vi "LV_n_UDP_clients.vi"() -> ()   [LabVIEW 2020]
panel:
  in  "Open Multi Ports":bool
  in  "Open Single Port":bool
  in  "Send Test Image":bool
  in  "h":i32=10 min=1 max=5000 step=1
  in  "w":i32=1 min=1 max=5000 step=1
  out "Elaps ms":u32
  in  "Send Image":bool
  out "Path to Python script":path
  in  "Stop":bool
  out "Answer":string
  in  "Ping":bool
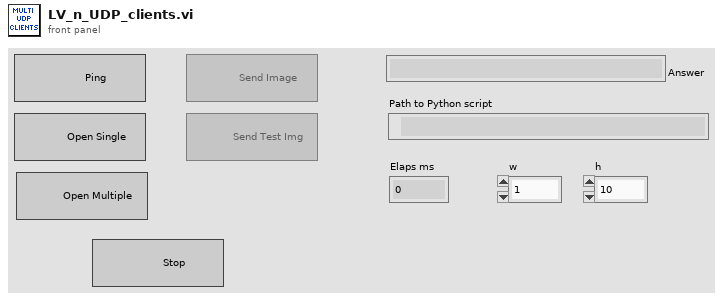
[diagram p1: front panel]
types:
  T1 = enum8{"Enabled", "Disabled", "Disabled and Grayed Out"}
  T2 = typedef "Image Type" = u32
  T3 = typedef "IMAQ Image.ctl" = refnum<image>
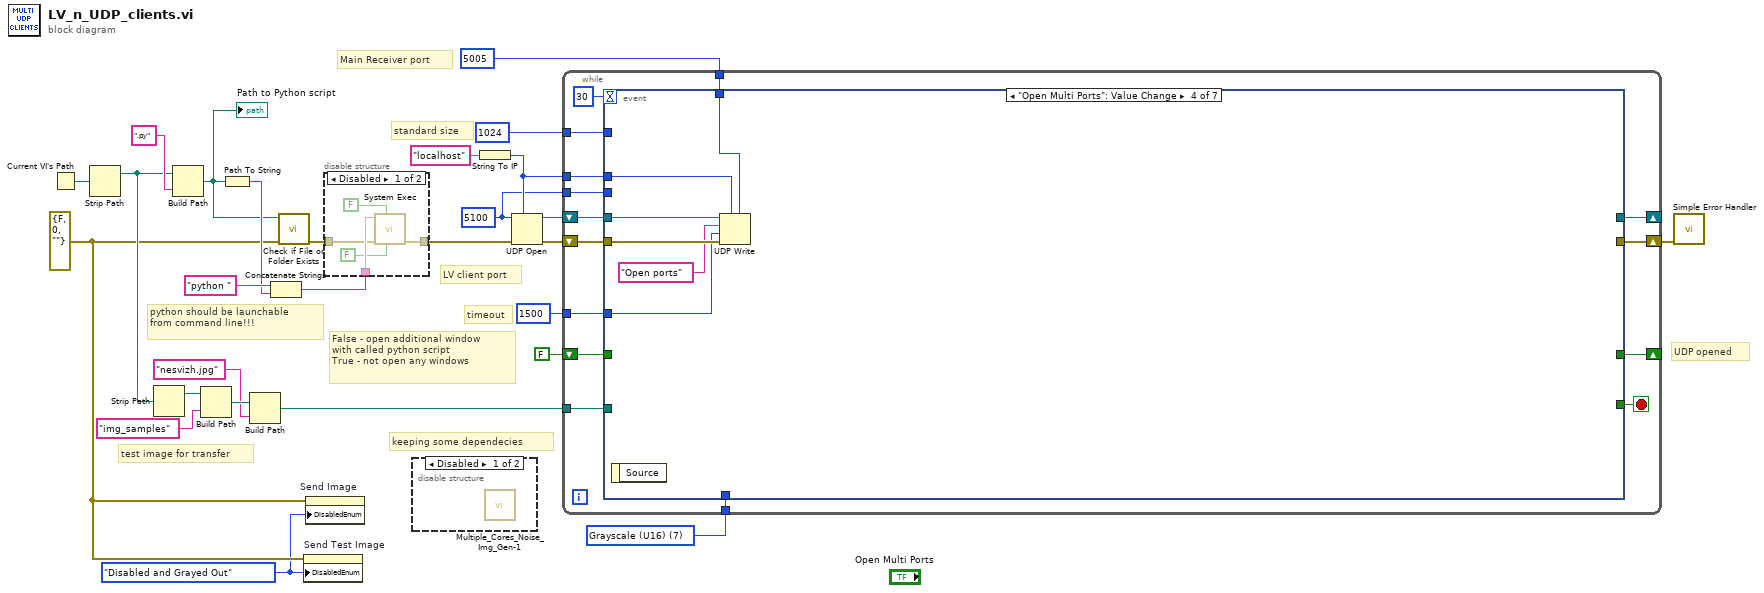
[diagram p0: block diagram]
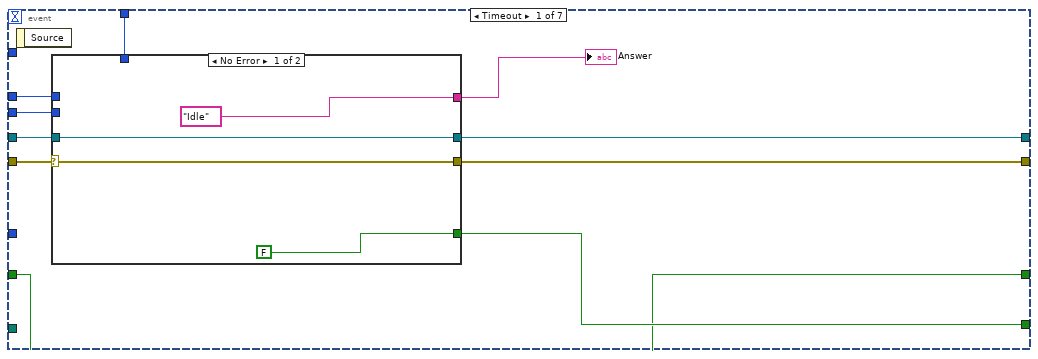
[diagram p4: hidden frame]
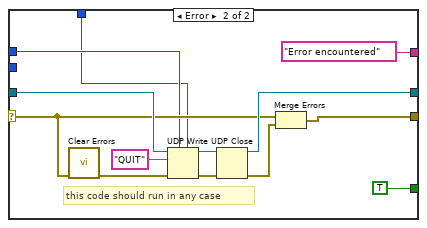
[diagram p5: hidden frame]
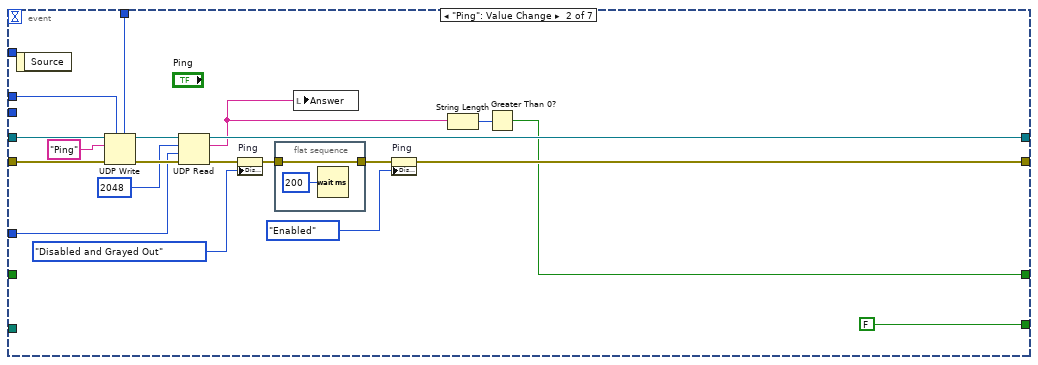
[diagram p6: hidden frame]
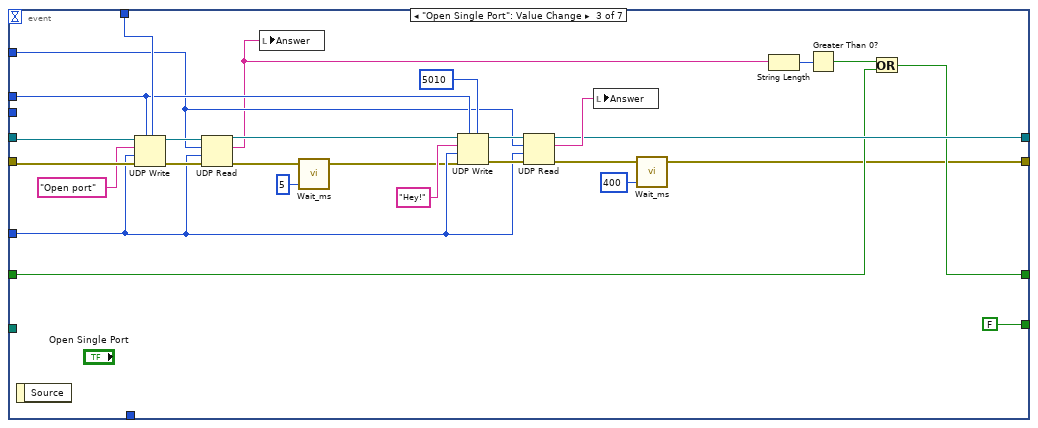
[diagram p7: hidden frame]
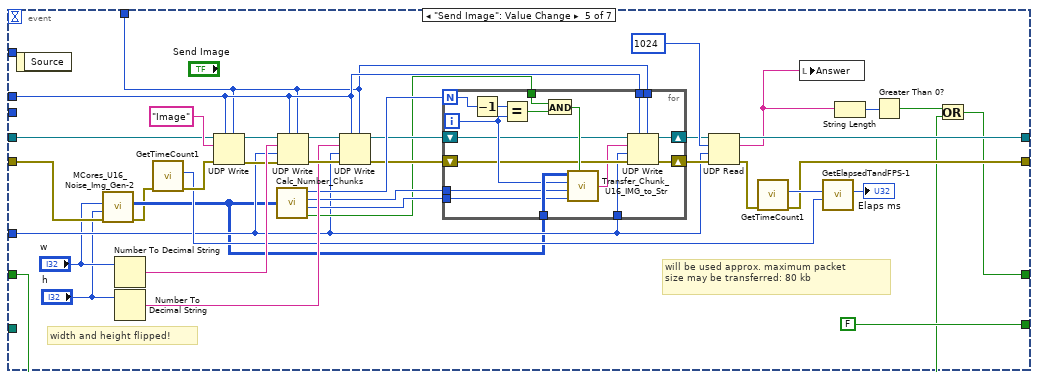
[diagram p8: hidden frame]
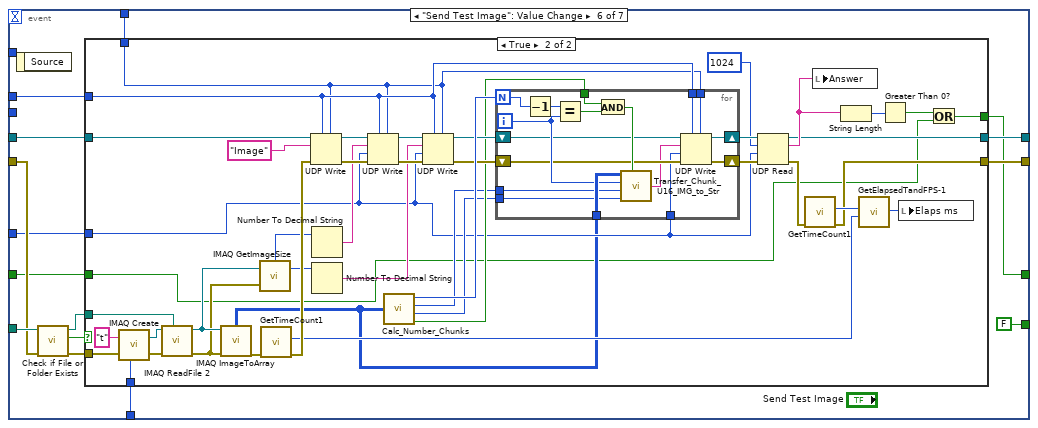
[diagram p9: hidden frame]
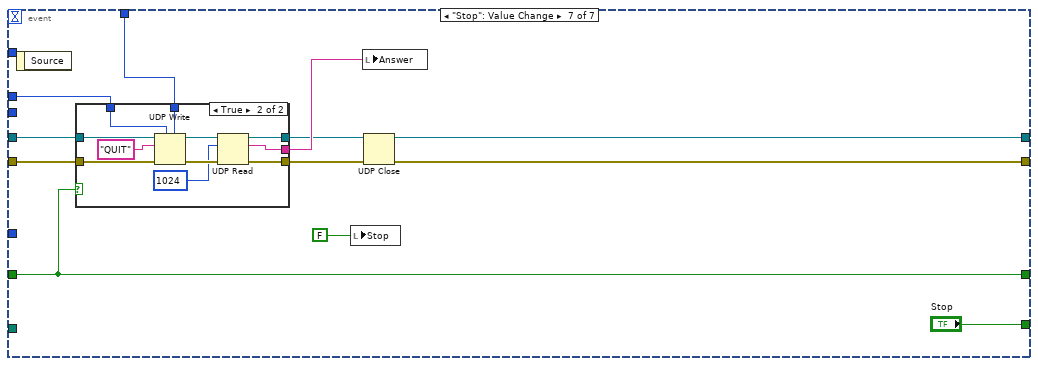
[diagram p11: hidden frame]
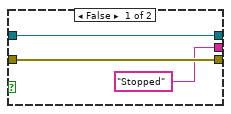
[diagram p12: hidden frame]
diagram:
  w3 = T1."Disabled and Grayed Out" ("Disabled")
  w5 = T2 7 items=["Grayscale (U8)", "Grayscale (I16)", "Grayscale (SGL)", "Complex (CSG)", "RGB (U32)", "HSL (U32)", "RGB (U64)", "Grayscale (U16)"] ("Image Type")
  w14 = u16 5100 ("remote port or service name")
  w4 = errorcluster {"status"=FALSE, "code"=0, "source"=""} ("error in (no error)")
  # "standard size"
  # "UDP opened"
  # "test image for transfer"
  # "keeping some dependecies"
  # "timeout"
  # "Main Receiver port"
  # "LV client port"
  # "False - open additional window\nwith called python script\nTrue - not open any windows"
  # "python should be launchable \nfrom command line!!!"
  n1 = Current VI's Path() -> (path=w26:path)
  n2 = Strip Path(path=w26) -> (stripped path=w11:path)  [unwired: 1 out]
  n3 = Strip Path(path=w11) -> (stripped path=w10:path)  [unwired: 1 out]
  n4 = Build Path(base path=w11, name or relative path=".py" ("string")) -> (appended path=w21:path)
  "Path to Python script" <- w21
  n5 = Build Path(base path=w10, name or relative path="img_samples" ("string")) -> (appended path=w8:path)
  n6 = Path To String(path=w21) -> (string=w22:string)
  n7 = Build Path(base path=w8, name or relative path="nesvizh.jpg" ("string")) -> (appended path=w6:path)
  n8 = Concatenate Strings("python " ("command line"), w22) -> (w24:string)
  n9 = call <vilib>:"Check if File or Folder Exists.vi"("error in (no error)"=w4, "path"=w21) -> ("error out"=w20:errorcluster)  [unwired: 7 in, 2 out]
  n10 = property on="Send Test Image" class="Bool"(error in=w4, "DisabledEnum"=w3) -> ()  [unwired: 1 in, 2 out]
  n11 = property on="Send Image" class="Bool"(error in=w4, "DisabledEnum"=w3) -> ()  [unwired: 1 in, 2 out]
  n12 = disable-structure shown="Disabled" {
    disable-tunnel: w24 -> [w32 _]
    disable-tunnel: [w31 w33] -> w19
    disable-tunnel: w20 -> [w29 w33]
    frame Disabled {
      n13 = call <vilib>:"System Exec.vi"("run minimized? (F)"=FALSE, "wait until completion? (T)"=FALSE, "error in (no error)"=w29, "command line"=w32) -> ("error out"=w31:errorcluster)  [unwired: 4 in, 3 out]
    }
    frame Enabled {
    }
  }
  n14 = disable-structure shown="Disabled" {
    frame Disabled {
      n15 = call "Multiple_Cores_Noise_Img_Gen-1.vi"() -> ()  [unwired: 10 in, 2 out]
    }
    frame Enabled {
    }
  }
  n16 = String To IP(1:"localhost" ("address")) -> (0:w15:u32)
  n17 = UDP Open(7:w15, 8:w19, 11:w14) -> (port=w17:refnum<k16>, 0:w18:errorcluster)  [unwired: 2 in, 1 out]
  n18 = while {
    shift-right: [w45] -> _
    shift-left: w17 -> [w46]
    shift-right: [w43] -> w27
    shift-left: w18 -> [w47]
    tunnel: w15 -> [w41]
    tunnel: w14 -> [w42]
    tunnel: u16 5005 ("remote port or service name") -> [w40]
    tunnel: 1500 -> [w39]
    tunnel: w6 -> [w38]
    tunnel: w5 -> [w37]
    shift-right: [w35] -> _
    shift-left: FALSE -> [w36]
    tunnel: 1024 -> [w34]
    stop <- w44 stop-if-true
    n19 = event shown="[3] \"Open Multi Ports\": Value Change" {
      selector: _ -> [_ _ _ _ _ _ _]
      dyn-events: _ -> [_ _ _ _ _ _ _]
      timeout: 30 -> [_ _ _ _ _ _ _]
      tunnel: [w54 FALSE ("Stop") FALSE ("Stop") _ FALSE ("Stop") FALSE ("Stop") "Stop"] -> w44
      tunnel: w47 -> [w58 w89 w125 w131 w141 w199 w272]
      tunnel: w46 -> [w57 w88 w124 w129 w168 w194 w273]
      tunnel: [w56 w84 w110 _ w162 w189 w274] -> w45
      tunnel: [w55 w91 w99 _ w154 w190 w275] -> w43
      tunnel: w42 -> [w52 _ _ _ _ _ _]
      tunnel: w41 -> [w51 w81 w118 w128 w143 w193 w268]
      tunnel: w40 -> [w50 w80 w122 w127 w142 w192 w267]
      tunnel: w39 -> [_ w79 w113 w126 w144 w191 _]
      tunnel: w38 -> [_ _ _ _ _ w200 _]
      tunnel: w37 -> [_ _ _ _ _ w195 _]
      tunnel: w36 -> [w49 _ w107 _ w133 w187 w266]
      tunnel: [w49 w76 w105 _ w132 w188 w266] -> w35
      tunnel: w34 -> [_ _ w112 _ _ _ _]
      event Timeout {
        n20 = event-data() -> ()  [unwired: 1 in, 1 out]
        n21 = case shown="No Error" w58 {
          selector: w58 -> [w61 w70]
          tunnel: [w62 w73] -> w56
          tunnel: w57 -> [w62 w72]
          tunnel: [w61 w71] -> w55
          tunnel: [FALSE ("Stop") TRUE ("Stop")] -> w54
          tunnel: ["Idle" ("Answer") "Error encountered" ("Answer")] -> w53
          tunnel: w52 -> [_ _]
          tunnel: w51 -> [_ w69]
          tunnel: w50 -> [_ w68]
          frame No Error {
          }
          frame Error {
            # "this code should run in any case"
            n22 = call <vilib>:"Clear Errors.vi"("error in (no error)"=w70) -> ("error out"=w67:errorcluster)  [unwired: 5 in, 1 out]
            n23 = UDP Write(address=w69, port or service name=w68, connection ID=w72, data in="QUIT", 8:w67) -> (error out=w66:errorcluster, 3:w64:refnum<k16>)  [unwired: 1 in]
            n24 = UDP Close(connection ID=w64, 8:w66) -> (connection ID out=w73:refnum<k16>, error out=w63:errorcluster)
            n25 = Merge Errors(w70, w63) -> (w71:errorcluster)
          }
        }
        "Answer" <- w53
      }
      event "Ping": Value Change {
        n26 = event-data() -> ()  [unwired: 1 in, 1 out]
        n27 = UDP Write(address=w81, port or service name=w80, connection ID=w88, data in="Ping", 8:w89) -> (error out=w86:errorcluster, 3:w85:refnum<k16>)  [unwired: 1 in]
        n28 = UDP Read(connection ID=w85, max size (548)=2048 ("bytes to read"), timeout ms (25000)=w79, 8:w86) -> (data out=w78:string, error out=w83:errorcluster, 3:w84:refnum<k16>)  [unwired: 2 out]
        n29 = property on="Ping" class="Bool"(error in=w83, "DisabledEnum"=T1."Disabled and Grayed Out" ("Disabled")) -> (error out=w94:errorcluster)  [unwired: 1 in, 1 out]
        n30 = flat-sequence {
          tunnel: w94 -> [w96]
          tunnel: [w96] -> w92
          frame #0 {
            n31 = Wait (ms)(milliseconds to wait=u32 200) -> ()  [unwired: 1 out]
          }
        }
        n32 = local write "Answer"(w78) -> ()
        n33 = property on="Ping" class="Bool"(error in=w92, "DisabledEnum"=T1."Enabled" ("Disabled")) -> (error out=w91:errorcluster)  [unwired: 1 in, 1 out]
        n34 = String Length(string=w78) -> (length=w77:i32)
        n35 = Greater Than 0?(x=w77) -> (x > 0?=w76:bool)
      }
      event "Open Single Port": Value Change {
        n36 = event-data() -> ()  [unwired: 1 in, 1 out]
        n37 = UDP Write(address=w118, port or service name=w122, connection ID=w124, data in="Open port", 8:w125, 9:w113) -> (error out=w120:errorcluster, 3:w121:refnum<k16>)
        n38 = UDP Read(connection ID=w121, max size (548)=w112, timeout ms (25000)=w113, 8:w120) -> (data out=w108:string, error out=w103:errorcluster, 3:w119:refnum<k16>)  [unwired: 2 out]
        n39 = local write "Answer"(w108) -> ()
        n40 = call "Wait_ms.vi"("[IN] Suspend ms"=u32 5, "error IN"=w103) -> ("error OUT"=w102:errorcluster)  [unwired: 3 in]
        n41 = UDP Write(address=w118, port or service name=u16 5010, connection ID=w119, data in="Hey!", 8:w102, 9:w113) -> (error out=w114:errorcluster, 3:w115:refnum<k16>)
        n42 = UDP Read(connection ID=w115, max size (548)=w112, timeout ms (25000)=w113, 8:w114) -> (data out=w111:string, error out=w100:errorcluster, 3:w110:refnum<k16>)  [unwired: 2 out]
        n43 = local write "Answer"(w111) -> ()
        n44 = call "Wait_ms.vi"("[IN] Suspend ms"=u32 400, "error IN"=w100) -> ("error OUT"=w99:errorcluster)  [unwired: 3 in]
        n45 = String Length(string=w108) -> (length=w109:i32)
        n46 = Greater Than 0?(x=w109) -> (x > 0?=w106:bool)
        n47 = Or(x=w106, y=w107) -> (x .or. y?=w105:bool)
      }
      event "Open Multi Ports": Value Change {
        n48 = event-data() -> ()  [unwired: 1 in, 1 out]
        n49 = UDP Write(address=w128, port or service name=w127, connection ID=w129, data in="Open ports", 8:w131, 9:w126) -> ()  [unwired: 2 out]
      }
      event "Send Image": Value Change {
        # "width and height flipped!"
        # "will be used approx. maximum packet \nsize may be transferred: 80 kb"
        n50 = event-data() -> ()  [unwired: 1 in, 1 out]
        n51 = call "MCores_U16_Noise_Img_Gen-2.vi"("error IN"=w141, "[IN] Width"="h", "[IN] Height"="w") -> ("error OUT"=w139:errorcluster, "[OUT] U16 Pixel Img"=w140:u16[][])  [unwired: 7 in]
        n52 = Number To Decimal String(number="w") -> (decimal integer string=w164:string)  [unwired: 1 in]
        n53 = Number To Decimal String(number="h") -> (decimal integer string=w161:string)  [unwired: 1 in]
        n54 = call "GetTimeCount1.vi"("error IN"=w139) -> ("error OUT"=w158:errorcluster, "[OUT] Timer Count"=w155:u32)  [unwired: 9 in]
        n55 = UDP Write(address=w143, port or service name=w142, connection ID=w168, data in="Image", 8:w158) -> (error out=w159:errorcluster, 3:w160:refnum<k16>)  [unwired: 1 in]
        n56 = call "Calc_Number_Chunks.vi"("[IN] U16 Pixel Img"=w140) -> ("[OUT] Number of chunks"=w151:i32, "[OUT] # rows single transfer"=w150:i32, "[OUT] # rows last transfer"=w149:i32, "[OUT] Not-equal last transfer"=w145:bool)
        n57 = UDP Write(address=w143, port or service name=w142, connection ID=w160, data in=w164, 8:w159, 9:w144) -> (error out=w167:errorcluster, 3:w166:refnum<k16>)
        n58 = UDP Write(address=w143, port or service name=w142, connection ID=w166, data in=w161, 8:w167, 9:w144) -> (error out=w147:errorcluster, 3:w148:refnum<k16>)
        n59 = for {
          N: w151 -> [w186]
          shift-right: [w176] -> w152
          shift-left: w147 -> [w177]
          tunnel: w140 -> [w184]
          tunnel: w150 -> [w179]
          tunnel: w149 -> [w178]
          shift-right: [w175] -> w146
          shift-left: w148 -> [w174]
          tunnel: w145 -> [w181]
          tunnel: w144 -> [w172]
          tunnel: w143 -> [w171]
          tunnel: w142 -> [w170]
          i -> [w182]
          n60 = Decrement(x=w186) -> (x-1=w185:i32)
          n61 = Equal?(x=w185, y=w182) -> (x = y?=w180:bool)
          n62 = And(x=w181, y=w180) -> (x .and. y?=w183:bool)
          n63 = call "Transfer_Chunk_U16_IMG_to_Str.vi"("[IN] U16 Pixel Img"=w184, "[IN] # of chunk"=w182, "[IN] # rows single transfer"=w179, "[IN] # rows last transfer"=w178, "[IN] Use remained rows"=w183) -> ("[OUT] Converted String"=w173:string)
          n64 = UDP Write(address=w171, port or service name=w170, connection ID=w174, data in=w173, 8:w177, 9:w172) -> (error out=w176:errorcluster, 3:w175:refnum<k16>)
        }
        n65 = UDP Read(connection ID=w146, max size (548)=1024 ("bytes to read"), timeout ms (25000)=w144, 8:w152) -> (data out=w135:string, error out=w157:errorcluster, 3:w162:refnum<k16>)  [unwired: 2 out]
        n66 = call "GetTimeCount1.vi"("error IN"=w157) -> ("error OUT"=w154:errorcluster, "[OUT] Timer Count"=w156:u32)  [unwired: 9 in]
        n67 = local write "Answer"(w135) -> ()
        n68 = call "GetElapsedTandFPS-1.vi"("[IN] Timer Count Before ALL [ms]"=w155, "[IN] Timer Count After ALL [ms]"=w156) -> ("[OUT] Elapsed time [ms]"=→"Elaps ms":u32)  [unwired: 3 in, 2 out]
        n69 = String Length(string=w135) -> (length=w136:i32)
        n70 = Greater Than 0?(x=w136) -> (x > 0?=w134:bool)
        n71 = Or(x=w134, y=w133) -> (x .or. y?=w132:bool)
      }
      event "Send Test Image": Value Change {
        n72 = event-data() -> ()  [unwired: 1 in, 1 out]
        n73 = call <vilib>:"Check if File or Folder Exists.vi"("error in (no error)"=w199, "path"=w200) -> ("error out"=w198:errorcluster, "file or folder exists?"=w197:bool, "dup path"=w196:path)  [unwired: 7 in]
        n74 = case shown="True" w197 {
          tunnel: w198 -> [w203 w248]
          tunnel: w196 -> [_ w243]
          tunnel: w195 -> [_ w247]
          tunnel: w194 -> [w204 w241]
          tunnel: w193 -> [_ w222]
          tunnel: w192 -> [_ w221]
          tunnel: w191 -> [_ w218]
          tunnel: [w203 w212] -> w190
          tunnel: [w204 w207] -> w189
          tunnel: [w202 w206] -> w188
          tunnel: w187 -> [w202 w205]
          frame False {
          }
          frame True {
            n75 = call "IMAQ Create"("Image Name"="t", "Image Type"=w247, "error in (no error)"=w248) -> ("New Image"=w244:T3, "error out"=w245:errorcluster)  [unwired: 2 in]
            n76 = call "IMAQ ReadFile 2"("File Path"=w243, "error in (no error)"=w245, "Image"=w244) -> ("error out"=w237:errorcluster, "Image Out"=w238:T3)  [unwired: 4 in, 3 out]
            n77 = call "IMAQ ImageToArray"("error in (no error)"=w237, "Image"=w238) -> ("error out"=w242:errorcluster, "Image Pixels (U8)"=w211:u8[][])  [unwired: 2 in, 3 out]
            n78 = call "IMAQ GetImageSize"("Image"=w238, "error in (no error)"=w237) -> ("Y Resolution"=w235:i32, "X Resolution"=w236:i32)  [unwired: 2 in, 1 out]
            n79 = call "GetTimeCount1.vi"("error IN"=w242) -> ("error OUT"=w240:errorcluster, "[OUT] Timer Count"=w215:u32)  [unwired: 9 in]
            n80 = UDP Write(address=w222, port or service name=w221, connection ID=w241, data in="Image", 8:w240) -> (error out=w234:errorcluster, 3:w233:refnum<k16>)  [unwired: 1 in]
            n81 = Number To Decimal String(number=w236) -> (decimal integer string=w232:string)  [unwired: 1 in]
            n82 = Number To Decimal String(number=w235) -> (decimal integer string=w229:string)  [unwired: 1 in]
            n83 = UDP Write(address=w222, port or service name=w221, connection ID=w233, data in=w232, 8:w234, 9:w218) -> (error out=w230:errorcluster, 3:w231:refnum<k16>)
            n84 = call "Calc_Number_Chunks.vi"("[IN] U16 Pixel Img"=w211) -> ("[OUT] Number of chunks"=w228:i32, "[OUT] # rows single transfer"=w224:i32, "[OUT] # rows last transfer"=w223:i32, "[OUT] Not-equal last transfer"=w225:bool)
            n85 = UDP Write(address=w222, port or service name=w221, connection ID=w231, data in=w229, 8:w230, 9:w218) -> (error out=w226:errorcluster, 3:w227:refnum<k16>)
            n86 = for {
              N: w228 -> [w265]
              shift-right: [w255] -> w220
              shift-left: w226 -> [w256]
              tunnel: w211 -> [w263]
              tunnel: w224 -> [w258]
              tunnel: w223 -> [w257]
              shift-right: [w254] -> w219
              shift-left: w227 -> [w253]
              tunnel: w225 -> [w260]
              tunnel: w218 -> [w251]
              tunnel: w222 -> [w250]
              tunnel: w221 -> [w249]
              i -> [w261]
              n87 = Decrement(x=w265) -> (x-1=w264:i32)
              n88 = Equal?(x=w264, y=w261) -> (x = y?=w259:bool)
              n89 = And(x=w260, y=w259) -> (x .and. y?=w262:bool)
              n90 = call "Transfer_Chunk_U16_IMG_to_Str.vi"("[IN] U16 Pixel Img"=w263, "[IN] # of chunk"=w261, "[IN] # rows single transfer"=w258, "[IN] # rows last transfer"=w257, "[IN] Use remained rows"=w262) -> ("[OUT] Converted String"=w252:string)
              n91 = UDP Write(address=w250, port or service name=w249, connection ID=w253, data in=w252, 8:w256, 9:w251) -> (error out=w255:errorcluster, 3:w254:refnum<k16>)
            }
            n92 = UDP Read(connection ID=w219, max size (548)=1024 ("bytes to read"), timeout ms (25000)=w218, 8:w220) -> (data out=w209:string, error out=w217:errorcluster, 3:w207:refnum<k16>)  [unwired: 2 out]
            n93 = call "GetTimeCount1.vi"("error IN"=w217) -> ("error OUT"=w212:errorcluster, "[OUT] Timer Count"=w216:u32)  [unwired: 9 in]
            n94 = local write "Answer"(w209) -> ()
            n95 = String Length(string=w209) -> (length=w210:i32)
            n96 = call "GetElapsedTandFPS-1.vi"("[IN] Timer Count Before ALL [ms]"=w215, "[IN] Timer Count After ALL [ms]"=w216) -> ("[OUT] Elapsed time [ms]"=w213:u32)  [unwired: 3 in, 2 out]
            n97 = Greater Than 0?(x=w210) -> (x > 0?=w208:bool)
            n98 = local write "Elaps ms"(w213) -> ()
            n99 = Or(x=w208, y=w205) -> (x .or. y?=w206:bool)
          }
        }
      }
      event "Stop": Value Change {
        n100 = event-data() -> ()  [unwired: 1 in, 1 out]
        n101 = case shown="True" w266 {
          tunnel: w273 -> [w280 w291]
          tunnel: w272 -> [w279 w290]
          tunnel: [w279 w286] -> w271
          tunnel: ["Stopped" ("data out") w285] -> w270
          tunnel: [w280 w284] -> w269
          tunnel: w268 -> [_ w282]
          tunnel: w267 -> [_ w281]
          frame False {
          }
          frame True {
            n102 = UDP Write(address=w282, port or service name=w281, connection ID=w291, data in="QUIT", 8:w290) -> (error out=w287:errorcluster, 3:w288:refnum<k16>)  [unwired: 1 in]
            n103 = UDP Read(connection ID=w288, max size (548)=1024 ("bytes to read"), 8:w287) -> (data out=w285:string, error out=w286:errorcluster, 3:w284:refnum<k16>)  [unwired: 1 in, 2 out]
          }
        }
        n104 = local write "Stop"(FALSE ("Stop")) -> ()
        n105 = local write "Answer"(w270) -> ()
        n106 = UDP Close(connection ID=w269, 8:w271) -> (connection ID out=w274:refnum<k16>, error out=w275:errorcluster)
      }
    }
  }
  n107 = call <vilib>:"Simple Error Handler.vi"("error in (no error)"=w27) -> ()  [unwired: 4 in, 5 out]
